vi "Inverse Kinematics (Trajectory).vi"(5 "max steps":i32=100, 7 "mask":dbl[](array[numeric]), 8 "error in (no error)":errorcluster, 9 "current joint positions":dbl[](array[numeric]), 10 "end effector trajectory":dbl[][][](array[numeric]), 11 "serial arm in":refnum<class "NI_Robotics_Serial Robot Arm.lvclass">) -> (0 "error out":errorcluster, 1 "steps taken":i32[](array[numeric]), 2 "joint position trajectory":dbl[][](array[numeric]), 3 "serial arm out":refnum<class "NI_Robotics_Serial Robot Arm.lvclass">)   [LabVIEW 2017, in "NI_Kinematics.lvlib"]
doc: "Computes the joint angles of a robotic arm given the location of the end effector relative to the arm base. Wire data to the <B>end effector transform</B> input to determine the polymorphic instance to use or manually select the instance.\n\n<B>.m file:</B> ikine"
uses:
  <vilib>/robotics/Kinematics/NI_Kinematics.lvlib
  <vilib>/robotics/Kinematics/Robot/NI_Robotics_Serial Robot Arm.lvclass
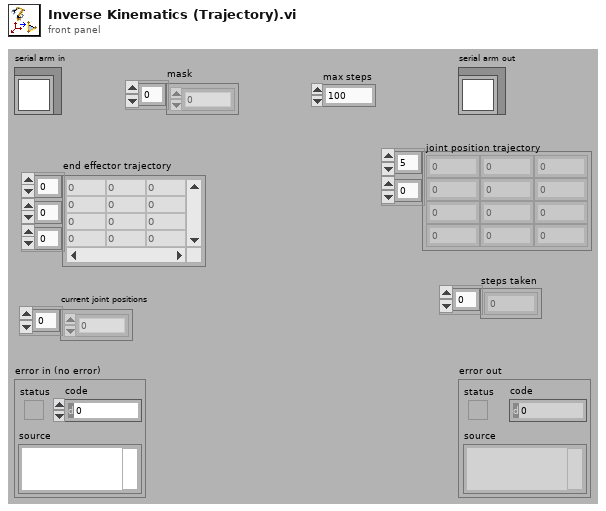
[diagram p1: front panel]
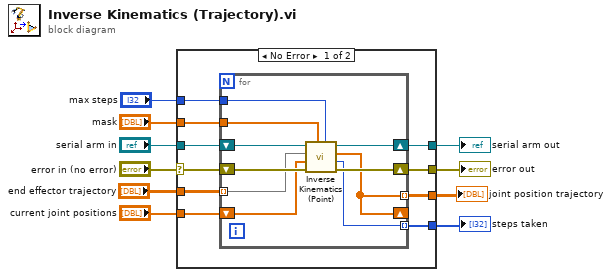
[diagram p0: block diagram]
diagram:
  n1 = case shown="No Error" "error in (no error)" {
    selector: "error in (no error)" -> [w19 w32]
    tunnel: [w15 w32] -> w9
    tunnel: [w14 w31] -> w7
    tunnel: "serial arm in" -> [w20 w31]
    tunnel: "end effector trajectory" -> [w18 _]
    tunnel: "mask" -> [w17 _]
    tunnel: "current joint positions" -> [w16 _]
    tunnel: [w13 _] -> w3
    tunnel: [w12 _] -> w2
    tunnel: "max steps" -> [w11 _]
    frame No Error {
      n2 = for {
        shift-right: [w26] -> w14
        shift-left: w20 -> [w30]
        shift-right: [w25] -> w15
        shift-left: w19 -> [w29]
        tunnel: w18 -> [w24] mode=indexing
        tunnel: w17 -> [w28]
        shift-right: [w23] -> _
        shift-left: w16 -> [w27]
        tunnel: [w23] -> w13 mode=indexing
        tunnel: [w22] -> w12 mode=indexing
        tunnel: w11 -> [w21]
        n3 = call <vilib>:"Inverse Kinematics (Point).vi"("max steps"=w21, "mask"=w28, "error in (no error)"=w29, "current joint positions"=w27, "end effector transform"=w24, "serial arm in"=w30) -> ("error out"=w25:errorcluster, "steps taken"=w22:i32, "joint positions"=w23:dbl[], "serial arm out"=w26:refnum<class "NI_Robotics_Serial Robot Arm.lvclass">)  [unwired: 2 out]
      }
    }
    frame Error {
    }
  }
  "error out" <- w9
  "serial arm out" <- w7
  "joint position trajectory" <- w3
  "steps taken" <- w2
